vi "Compute New Timeout - EXAMPLE 01.vi"   [LabVIEW 2009]
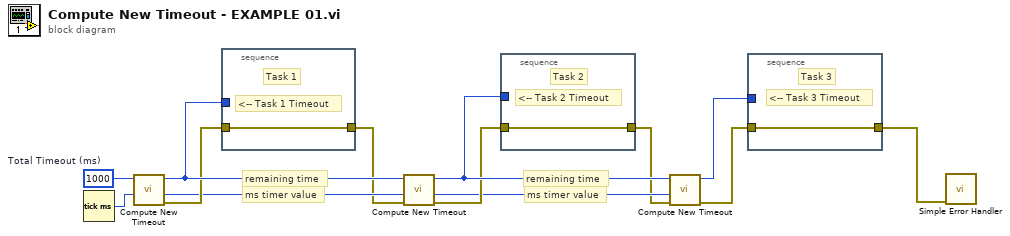
[diagram p0: block diagram]
diagram:
  w11 = 1000  # Total Timeout (ms)
  # "remaining time"
  # "remaining time"
  # "ms timer value"
  # "ms timer value"
  n1 = Tick Count (ms)() -> (millisecond timer value=w10:u32)
  n2 = call "Compute New Timeout.vi"("millisecond timer value (previous)"=w10, "timeout in ms"=w11) -> ("error out"=w12:errorcluster, "millisecond timer value (now)"=w9:u32, "timeout in ms (new)"=w13:i32)  [unwired: 7 in]
  n3 = stacked-sequence {
    tunnel: w13 -> [_]
    tunnel: w12 -> [w14]
    tunnel: [w14] -> w8
    frame #0 {
      # "<-- Task 1 Timeout"
      # "Task 1"
    }
  }
  n4 = call "Compute New Timeout.vi"("error in (no error)"=w8, "millisecond timer value (previous)"=w9, "timeout in ms"=w13) -> ("error out"=w6:errorcluster, "millisecond timer value (now)"=w5:u32, "timeout in ms (new)"=w7:i32)  [unwired: 6 in]
  n5 = stacked-sequence {
    tunnel: w6 -> [w15]
    tunnel: [w15] -> w4
    tunnel: w7 -> [_]
    frame #0 {
      # "<-- Task 2 Timeout"
      # "Task 2"
    }
  }
  n6 = call "Compute New Timeout.vi"("error in (no error)"=w4, "millisecond timer value (previous)"=w5, "timeout in ms"=w7) -> ("error out"=w2:errorcluster, "timeout in ms (new)"=w3:i32)  [unwired: 6 in, 1 out]
  n7 = stacked-sequence {
    tunnel: w2 -> [w16]
    tunnel: [w16] -> w1
    tunnel: w3 -> [_]
    frame #0 {
      # "<-- Task 3 Timeout"
      # "Task 3"
    }
  }
  n8 = call <vilib>:"Simple Error Handler.vi"("error in (no error)"=w1) -> ()  [unwired: 4 in, 5 out]
